vi "Load Scan.vi"(8 "error in (no error)":errorcluster, 11 "XML File Path":path) -> (0 "error out":errorcluster, 3 "Scan Driver out":refnum<class "Scan Driver.lvclass">)   [LabVIEW 2017, in "Scan Driver.lvclass"]
doc: "Unflattens a Scan Driver instance from the specified XML file. If an error occurs, returns the class default object."
uses:
  Scan Driver.lvclass
  Scanner List.ctl
  Reader List.ctl
  Scan Driver.lvclass/Scan Driver.ctl
  Readers/LCD Reader/LCD Reader.lvclass
  C:/LabVIEW-programs/Readers/Reader/Reader.lvclass
  Settings Panel.vi
  <vilib>/Utility/file.llb/Read From Spreadsheet File (I64).vi
  File IO/File IO.lvclass
  Instruments/LCD/LCD Retarder.lvclass
  Scanners/Scanner/Scanner.lvclass
  Readers/Reader/Reader.lvclass
  <vilib>/Utility/xml.llb/Read From XML File(string).vi
panel:
  in  "Reader List":T1
  in  "Scanner List":T2
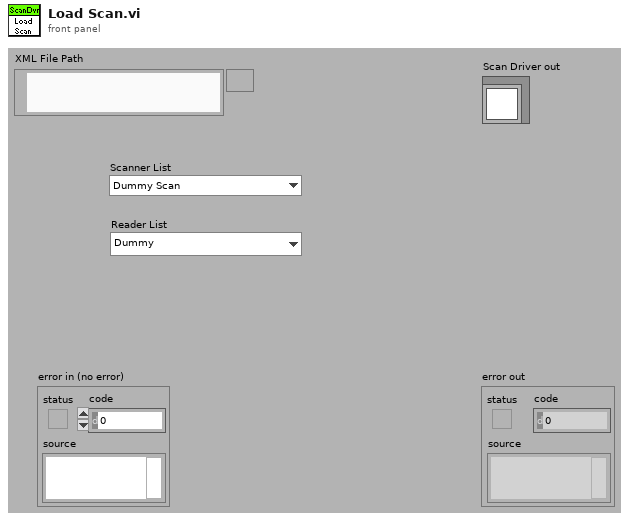
[diagram p1: front panel]
types:
  T1 = typedef "Scan Driver.lvclass/Reader List.ctl" = enum16{"Dummy", "Cryostat Temperature", "DAQmx Analog", "Lockin SR830", "Multimeter", "Photon Counter", "Power Meter", "Temperature Control"}
  T2 = typedef "Scan Driver.lvclass/Scanner List.ctl" = enum16{"Dummy Scan", "Analog Output Scan", "Function Gen Scan", "Magnetic Field Lakeshore", "Magnetic Field Lakeshore Continuous", "Magnetic Field Oxford", "Magnetic Field Oxford Continuous", "Magna Current Scan", "Magna Voltage Scan", "Microwave Freq Scan", "Pulse Gen Scan", "Pulse Gen Basic Scan", "Translation Stage Dual", "Translation Stage Coarse", "Translation Stage Fine", "Wavelength", "Wavelength Digikröm", "Wavelength ActiveX", "None"}
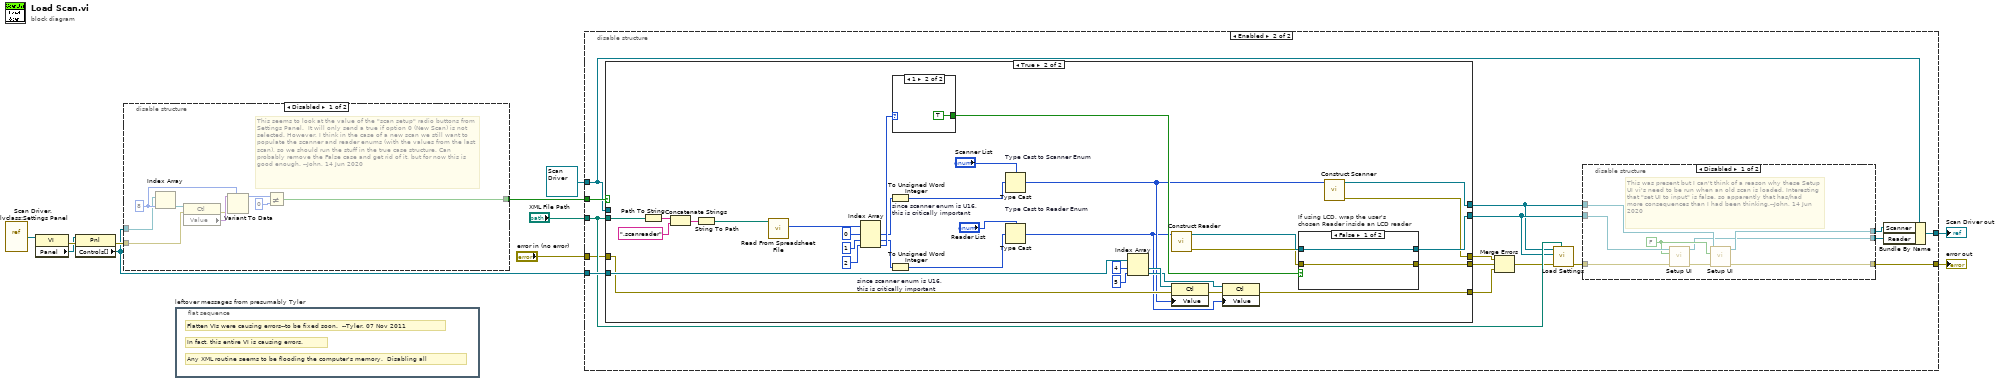
[diagram p0: block diagram]
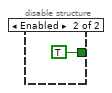
[diagram p2: hidden frame]
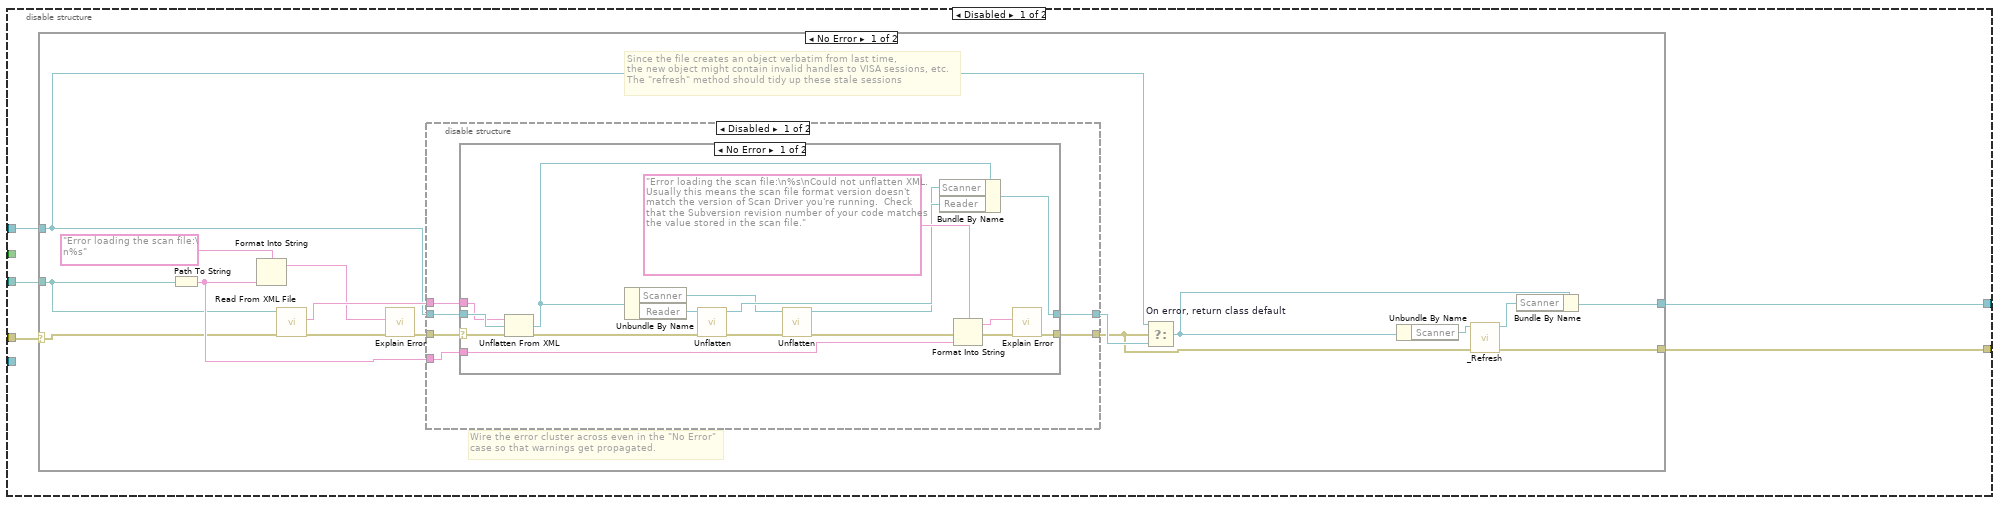
[diagram p3: hidden frame]
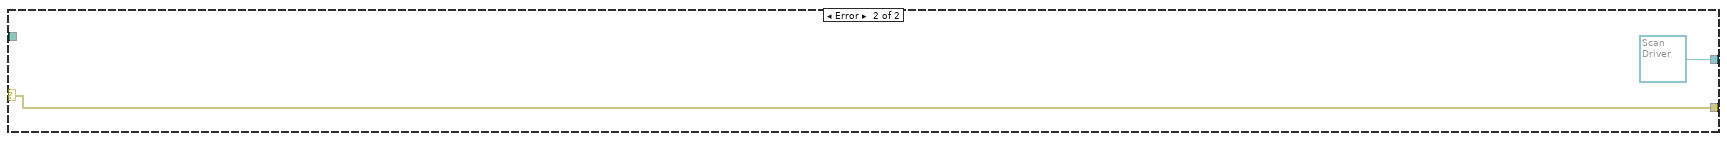
[diagram p6: hidden frame]
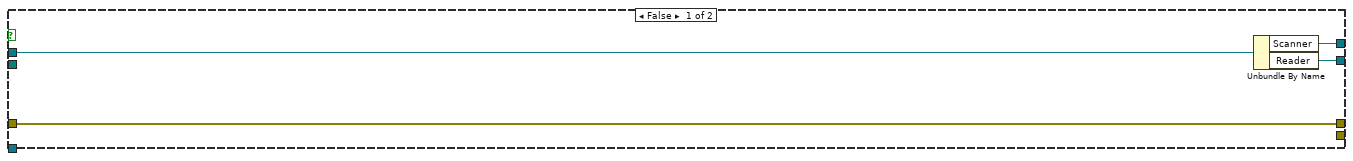
[diagram p8: hidden frame]
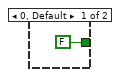
[diagram p9: hidden frame]
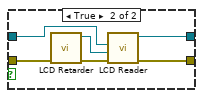
[diagram p10: hidden frame]
diagram:
  n1 = vi-ref "Scan Driver.lvclass:Settings Panel.vi"() -> (w3:refnum<vi>)
  n2 = property class="VI"(reference=w3) -> (error out=w6:errorcluster, "Panel"=w4:refnum<vi>)  [unwired: 1 in, 1 out]
  n3 = property class="Pnl"(reference=w4, error in=w6) -> (error out=w5:errorcluster, "Controls[]"=w2:refnum<vi>[])  [unwired: 1 out]
  n4 = disable-structure shown="Disabled" {
    disable-tunnel: w5 -> [w20 _]
    disable-tunnel: w2 -> [w15 _]
    disable-tunnel: [w13 TRUE] -> w1
    frame Disabled {
      w16 = 8 ("index")
      # "This seems to look at the value of the \"scan setup\" radio buttons from Settings Panel.  It will only send a true if option 0 (New Scan) is not selected. However, I think in the case of a new scan we still want to populate the scanner and reader enums (with the values from the last scan), so we should run the stuff in the true case structure. Can probably remove the False case and get rid of it, but for now this is good enough. --John, 14 Jun 2020"
      n5 = Index Array(array=w15, index=w16) -> (element=w19:refnum<vi>)
      n6 = property class="Ctl"(reference=w19, error in=w20) -> (error out=w17:errorcluster, "Value"=w18:variant)  [unwired: 1 out]
      n7 = Variant To Data(error in=w17, type=w16, Variant=w18) -> (data=w14:i32)  [unwired: 1 out]
      n8 = Not Equal?(x=w14, y=0) -> (x != y?=w13:bool)
    }
    frame Enabled {
    }
  }
  n9 = flat-sequence "leftover messages from presumably Tyler" {
    frame #0 {
      # "Flatten VIs were causing errors--to be fixed soon.  --Tyler, 07 Nov 2011"
      # "Any XML routine seems to be flooding the computer's memory.  Disabling all"
      # "In fact, this entire VI is causing errors."
    }
  }
  n10 = disable-structure shown="Enabled" {
    disable-tunnel: "error in (no error)" -> [w26 w83]
    disable-tunnel: [w25 w72] -> w10
    disable-tunnel: [w24 w78] -> w9
    disable-tunnel: "XML File Path" -> [w23 w84]
    disable-tunnel: refnum<class "Scan Driver.lvclass"> refnum ("Scan Driver out") -> [w22 w86]
    disable-tunnel: w1 -> [_ w87]
    disable-tunnel: w2 -> [_ w85]
    frame Disabled {
      n11 = case shown="No Error" w26 {
        selector: w26 -> [w36 w71]
        tunnel: [w30 w71] -> w25
        tunnel: [w34 refnum<class "Scan Driver.lvclass"> refnum ("Scan Driver out")] -> w24
        tunnel: w23 -> [w29 _]
        tunnel: w22 -> [w27 _]
        frame No Error {
          # "Since the file creates an object verbatim from last time,\nthe new object might contain invalid handles to VISA sessions, etc.\nThe \"refresh\" method should tidy up these stale sessions"
          # "Wire the error cluster across even in the \"No Error\"\ncase so that warnings get propagated."
          n12 = Path To String(path=w29) -> (string=w39:string)
          n13 = Format Into String(format string="Error loading the scan file:\n%s" ("error message (\"\")"), w39) -> (resulting string=w31:string)  [unwired: 2 in, 1 out]
          n14 = call-poly <vilib>:"Read From XML File.vi"("error in (no error)"=w36, "XML File Path"=w29) -> ("error out"=w28:errorcluster, "XML Elements"=w41:string)  [unwired: 8 out]
          n15 = call "Explain Error.vi"("error in"=w28, "Explanation"=w31) -> ("error out"=w32:errorcluster)  [unwired: 9 out]
          n16 = disable-structure shown="Disabled" {
            disable-tunnel: [w48 w68] -> w42
            disable-tunnel: w27 -> [w47 w68]
            disable-tunnel: w41 -> [w46 _]
            disable-tunnel: w39 -> [w45 _]
            disable-tunnel: [w44 w69] -> w33
            disable-tunnel: w32 -> [w43 w69]
            frame Disabled {
              n17 = case shown="No Error" w43 {
                selector: w43 -> [w63 w67]
                tunnel: [w58 w66] -> w48
                tunnel: w47 -> [w65 w66]
                tunnel: w46 -> [w64 _]
                tunnel: [w59 w67] -> w44
                tunnel: w45 -> [w61 _]
                frame No Error {
                  n18 = Unflatten From XML(xml string=w64, type=w65, error in (no error)=w63) -> (value=w57:refnum<class "Scan Driver.lvclass">, error out=w56:errorcluster)
                  n19 = Unbundle By Name(w57) -> ("Scanner"=w50:refnum<class "Scanner.lvclass">, "Reader"=w53:refnum<class "Reader.lvclass">)
                  n20 = call-dynamic "Unflatten.vi"("error in (no error)"=w56, "Reader in"=w53) -> ("error out"=w49:errorcluster, "Reader out"=w52:refnum<class "Reader.lvclass">)  [unwired: 8 in]
                  n21 = call-dynamic "Unflatten.vi"("error in (no error)"=w49, "Scanner in"=w50) -> ("error out"=w55:errorcluster, "Scanner out"=w51:refnum<class "Scanner.lvclass">)  [unwired: 8 in]
                  n22 = Bundle By Name(cluster=w57, "Scanner"=w51, "Reader"=w52) -> (w58:refnum<class "Scan Driver.lvclass">)
                  n23 = Format Into String(format string="Error loading the scan file:\n%s\nCould not unflatten XML.  Usually this means the scan file format version doesn't match the version of Scan Driver you're running.  Check that the Subversion revision number of your code matches the value stored in the scan file.", error in=w55, w61) -> (resulting string=w60:string, error out=w54:errorcluster)  [unwired: 1 in]
                  n24 = call "Explain Error.vi"("error in"=w54, "Explanation"=w60) -> ("error out"=w59:errorcluster)  [unwired: 9 out]
                }
                frame Error {
                }
              }
            }
            frame Enabled {
            }
          }
          n25 = Select "On error, return class default"(t=w27, s=w33, f=w42) -> (s? t:f=w35:refnum<class "Scan Driver.lvclass">)
          n26 = Unbundle By Name(w35) -> ("Scanner"=w38:refnum<class "Scanner.lvclass">)
          n27 = call-dynamic "_Refresh.vi"("error in (no error)"=w33, "Scanner in"=w38) -> ("error out"=w30:errorcluster, "Scanner out"=w37:refnum<class "Scanner.lvclass">)  [unwired: 8 out]
          n28 = Bundle By Name(cluster=w35, "Scanner"=w37) -> (w34:refnum<class "Scan Driver.lvclass">)
        }
        frame Error {
        }
      }
    }
    frame Enabled {
      n29 = case shown="True" w87 {
        tunnel: w86 -> [w102 _]
        tunnel: [w101 w109] -> w75
        tunnel: [w100 w124] -> w77
        tunnel: w85 -> [_ w122]
        tunnel: w84 -> [_ w135]
        tunnel: w83 -> [w99 w117]
        tunnel: [w99 w108] -> w82
        tunnel: [_ w123] -> w81
        tunnel: [_ w115] -> w79
        frame False {
          n30 = Unbundle By Name(w102) -> ("Scanner"=w101:refnum<class "Scanner.lvclass">, "Reader"=w100:refnum<class "Reader.lvclass">)
        }
        frame True {
          n31 = Path To String(path=w135) -> (string=w133:string)
          n32 = Concatenate Strings(w133, ".scanreader") -> (w132:string)
          n33 = String To Path(string=w132) -> (path=w131:path)
          n34 = call-poly <vilib>:"Read From Spreadsheet File.vi"("file path (dialog if empty)"=w131) -> ("first row"=w130:i64[])  [unwired: 6 in, 4 out]
          n35 = Index Array(array=w130, index #1=0 ("index"), index #2=1 ("index"), index #3=2 ("index")) -> (element #1=w114:i64, element #2=w111:i64, element #3=w126:i64)
          n36 = To Unsigned Word Integer "since scanner enum is U16, \nthis is critically important"(number=w114) -> (unsigned 16bit integer=w104:u16)
          n37 = To Unsigned Word Integer "since scanner enum is U16, \nthis is critically important"(number=w111) -> (unsigned 16bit integer=w103:u16)
          n38 = case shown="1" w126 {
            tunnel: [FALSE TRUE] -> w125
            frame 0, Default {
            }
            frame 1 {
            }
          }
          n39 = Type Cast "Type Cast to Scanner Enum"(type="Scanner List", x=w104) -> (*(type *) &x=w110:T2)
          n40 = Type Cast "Type Cast to Reader Enum"(type="Reader List", x=w103) -> (*(type *) &x=w107:T1)
          n41 = Index Array(array=w122, index #1=4 ("index"), index #2=5 ("index")) -> (element #1=w119:refnum<vi>, element #2=w118:refnum<vi>)
          n42 = call "Construct Reader.vi"("Reader Enum in"=w107) -> ("error out"=w105:errorcluster, "Reader out"=w106:refnum<class "Reader.lvclass">)  [unwired: 9 in]
          n43 = property class="Ctl"(reference=w119, error in=w117, "Value"=w110) -> (error out=w116:errorcluster)  [unwired: 1 out]
          n44 = property class="Ctl"(reference=w118, error in=w116, "Value"=w107) -> (error out=w115:errorcluster)  [unwired: 1 out]
          n45 = case "If using LCD, wrap the user's \nchosen Reader inside an LCD reader" shown="False" w125 {
            tunnel: w106 -> [w138 w142]
            tunnel: w105 -> [w139 w143]
            tunnel: [w139 w140] -> w123
            tunnel: [w138 w141] -> w124
            frame False {
            }
            frame True {
              n46 = call "LCD Retarder.vi"("error in"=w143) -> ("errorOUT"=w144:errorcluster, "LCD out"=w145:refnum<class "LCD Retarder.lvclass">)  [unwired: 9 out]
              n47 = call "LCD Reader.vi"("error in (no error)"=w144, "LCD Retarder in"=w145, "Reader.lvclass"=w142) -> ("error out"=w140:errorcluster, "LCD Reader out"=w141:refnum<class "LCD Reader.lvclass">)  [unwired: 2 in, 5 out]
            }
          }
          n48 = call "Construct Scanner.vi"("Scanner Enum In"=w110) -> ("error out"=w108:errorcluster, "Scanner out"=w109:refnum<class "Scanner.lvclass">)  [unwired: 9 in]
        }
      }
      n49 = Merge Errors(w82, w81, w79) -> (w80:errorcluster)
      n50 = call "Load Settings.vi"("Path"=w84, "error in (no error)"=w80, "Reader Object"=w77, "Scanner Object"=w75) -> ("error out"=w76:errorcluster)  [unwired: 7 in]
      n51 = disable-structure shown="Disabled" {
        disable-tunnel: w77 -> [w95 w98]
        disable-tunnel: w76 -> [w94 w96]
        disable-tunnel: w75 -> [w93 w97]
        disable-tunnel: [w90 w96] -> w72
        disable-tunnel: [w89 w97] -> w74
        disable-tunnel: [w88 w98] -> w73
        frame Disabled {
          w92 = FALSE
          # "This was present but I can't think of a reason why these Setup UI vi's need to be run when an old scan is loaded. Interesting that \"set UI to input\" is false, so apparently that has/had more consequences than I had been thinking.--John, 14 Jun 2020"
          n52 = call-dynamic "Setup UI.vi"("error in (no error)"=w94, "Set UI to input? (F)"=w92, "Reader in"=w95) -> ("error out"=w91:errorcluster, "Reader out"=w88:refnum<class "Reader.lvclass">)  [unwired: 1 in, 6 out]
          n53 = call-dynamic "Setup UI.vi"("error in (no error)"=w91, "Set UI to input? (F)"=w92, "Scanner in"=w93) -> ("error out"=w90:errorcluster, "Scanner out"=w89:refnum<class "Scanner.lvclass">)  [unwired: 7 out]
        }
        frame Enabled {
        }
      }
      n54 = Bundle By Name(cluster=w86, "Scanner"=w74, "Reader"=w73) -> (w78:refnum<class "Scan Driver.lvclass">)
    }
  }
  "error out" <- w10
  "Scan Driver out" <- w9
